vi "Check Status.vi"(8 "error in (no error)":errorcluster, 11 "Cryostat in":refnum<class "Cryostat.lvclass">) -> (0 "error out":errorcluster, 1 "Status":string, 2 "Ready?":bool, 3 "Cryostat out":refnum<class "Cryostat.lvclass">)   [LabVIEW 2023, in "Cryostat.lvclass"]
doc: "(Dynamic) Check if the instrument is powered on and update its member fields with the instrument's current status. Optionally return a text status message."
uses:
  Cryostat.lvclass
  Cryostat.lvclass/Cryostat.ctl
  Utility Classes/Readable/Readable.lvclass
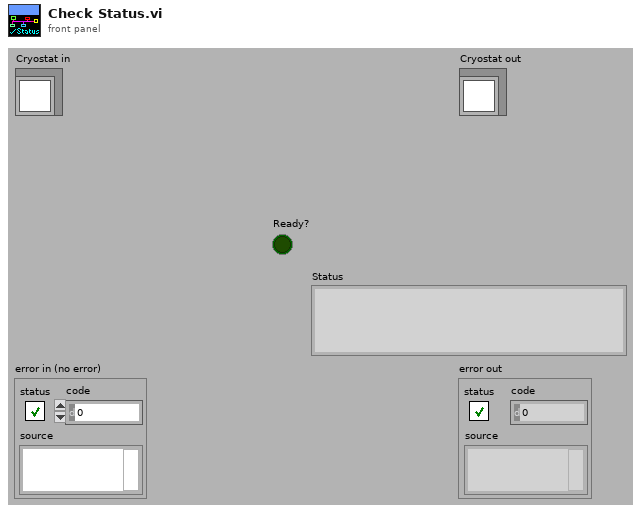
[diagram p1: front panel]
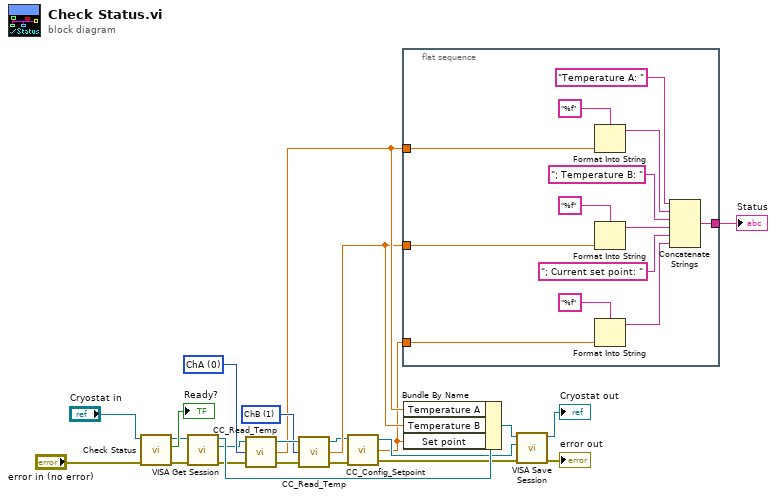
[diagram p0: block diagram]
diagram:
  w10 = u8 1 items=["ChA", "ChB", "ChC", "ChD"] ("Input")
  w11 = u8 0 items=["ChA", "ChB", "ChC", "ChD"] ("Input")
  n1 = call-parent "Check Status.vi"("error in (no error)"="error in (no error)", "Instrument in"="Cryostat in") -> ("error out"=w18:errorcluster, "Ready?"=→"Ready?":bool, "Instrument out"=w19:refnum<class "Cryostat.lvclass">)  [unwired: 6 in, 1 out]
  n2 = call-dynamic "VISA Get Session.vi"("error in (no error)"=w18, "Instrument.lvclass in"=w19) -> ("error out"=w14:errorcluster, "VISA Resource Name"=w1:refnum<visa-resource-name>, "Instrument.lvclass out"=w16:refnum<class "Cryostat.lvclass">)  [unwired: 7 out]
  n3 = call "CC_Read_Temp.vi"("error in (no error)"=w14, "Input"=w11, "VISA In"=w1) -> ("error out"=w13:errorcluster, "Temperature"=w9:dbl, "VISA Out"=w12:refnum<visa-resource-name>)
  n4 = call "CC_Read_Temp.vi"("error in (no error)"=w13, "Input"=w10, "VISA In"=w12) -> ("error out"=w4:errorcluster, "Temperature"=w8:dbl, "VISA Out"=w6:refnum<visa-resource-name>)
  n5 = call "CC_Config_Setpoint.vi"("error in (no error)"=w4, "VISA In"=w6) -> ("error out"=w3:errorcluster, "Set Point Returned"=w2:sgl, "VISA Out"=w5:refnum<visa-resource-name>)  [unwired: 2 in]
  n6 = flat-sequence {
    tunnel: [w36] -> w7
    tunnel: w8 -> [w30]
    tunnel: w9 -> [w31]
    tunnel: w2 -> [w26]
    frame #0 {
      n7 = Format Into String(format string="%f", w31) -> (resulting string=w29:string)  [unwired: 2 in, 1 out]
      n8 = Format Into String(format string="%f", w30) -> (resulting string=w28:string)  [unwired: 2 in, 1 out]
      n9 = Format Into String(format string="%f", w26) -> (resulting string=w24:string)  [unwired: 2 in, 1 out]
      n10 = Concatenate Strings("Temperature A: " ("string"), w29, "; Temperature B: " ("string"), w28, "; Current set point: " ("string"), w24) -> (w36:string)
    }
  }
  n11 = Bundle By Name(cluster=w16, "Temperature A"=w9, "Temperature B"=w8, "Set point"=w2) -> (w15:refnum<class "Cryostat.lvclass">)
  n12 = call-dynamic "VISA Save Session.vi"("error in (no error)"=w3, "VISA Resource Name"=w5, "Instrument.lvclass in"=w15) -> ("error out"=→"error out":errorcluster, "Instrument.lvclass out"=→"Cryostat out":refnum<class "Cryostat.lvclass">)  [unwired: 7 out]
  "Status" <- w7
